vi "Update Enclosed Area.vi"(10 "Start Vectors":T1, 11 "Map in":refnum<class "Maze.lvclass">) -> (3 "Map out":refnum<class "Maze.lvclass">)   [LabVIEW 2020, in "Maze.lvclass"]
uses:
  Maze.lvclass
  Position.ctl
  Maze.lvclass/Maze.ctl
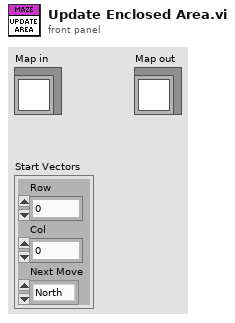
[diagram p1: front panel]
types:
  T1 = typedef "Maze.lvclass/Position.ctl" = cluster{"Row":u64, "Col":u64, "Next Move":enum16{"North", "East", "South", "West", "Halt"}}
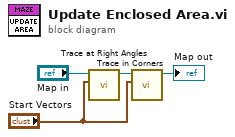
[diagram p0: block diagram]
diagram:
  n1 = call "Trace at Right Angles.vi"("Start Vectors"="Start Vectors", "Map in"="Map in") -> ("Map out"=w4:refnum<class "Maze.lvclass">)  [unwired: 9 in]
  n2 = call "Trace in Corners.vi"("Start Vectors"="Start Vectors", "Map in"=w4) -> ("Map out"=→"Map out":refnum<class "Maze.lvclass">)  [unwired: 9 in]
